vi "Read Network.vi"(8 "error in (no error)":errorcluster, 11 "Sensor Engine Datas in":T1[](array[typedef])) -> (0 "error out":errorcluster, 1 "signal data":dbl[](array[numeric]), 3 "Sensor Engine Datas out":T1[](array[typedef]))   [LabVIEW 2023, in "MM.lvlib"]
uses:
  MM.lvlib
  Sensor Engine Data.ctl
  DataContainer/DataContainer.lvclass
  Shared/Protocol.ctl
  <vilib>/xnet/xnet.llb/XNET Convert (Frame FlexRay to Signal).vi
  Shared/Vires VTD Shared.lvlib
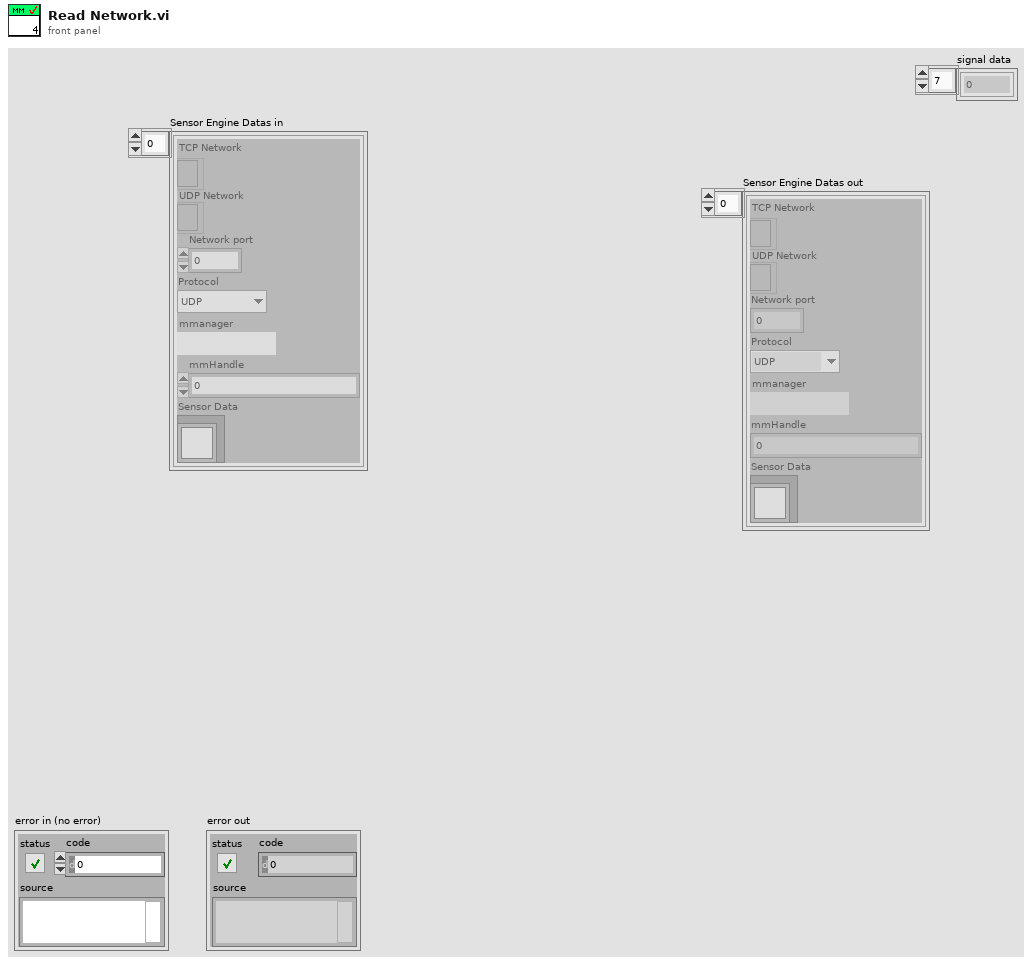
[diagram p1: front panel]
types:
  T1 = typedef "MM.lvlib/Sensor Engine Data.ctl" = cluster{"TCP Network":refnum<k5>, "UDP Network":refnum<k16>, "Network port":i32, "Protocol":T2, "mmanager":path, "mmHandle":u64, "Sensor Data":refnum<class "DataContainer.lvclass">}
  T2 = typedef "Vires VTD Shared.lvlib/Protocol.ctl" = enum16{"UDP", "TCP"}
  T3 = enum16{"Standard", "Buffered", "CRLF", "Immediate"}
  T4 = typedef "XNET Frame FlexRay.ctl" = cluster{"timestamp":timestamp, "payload":u8[], "slot":u16, "type":T5, "cycle count":u8, "startup?":bool, "sync?":bool, "preamble?":bool, "ch A":bool, "ch B":bool, "echo?":bool}
  T5 = typedef "XNET Frame Type FlexRay.ctl" = u8
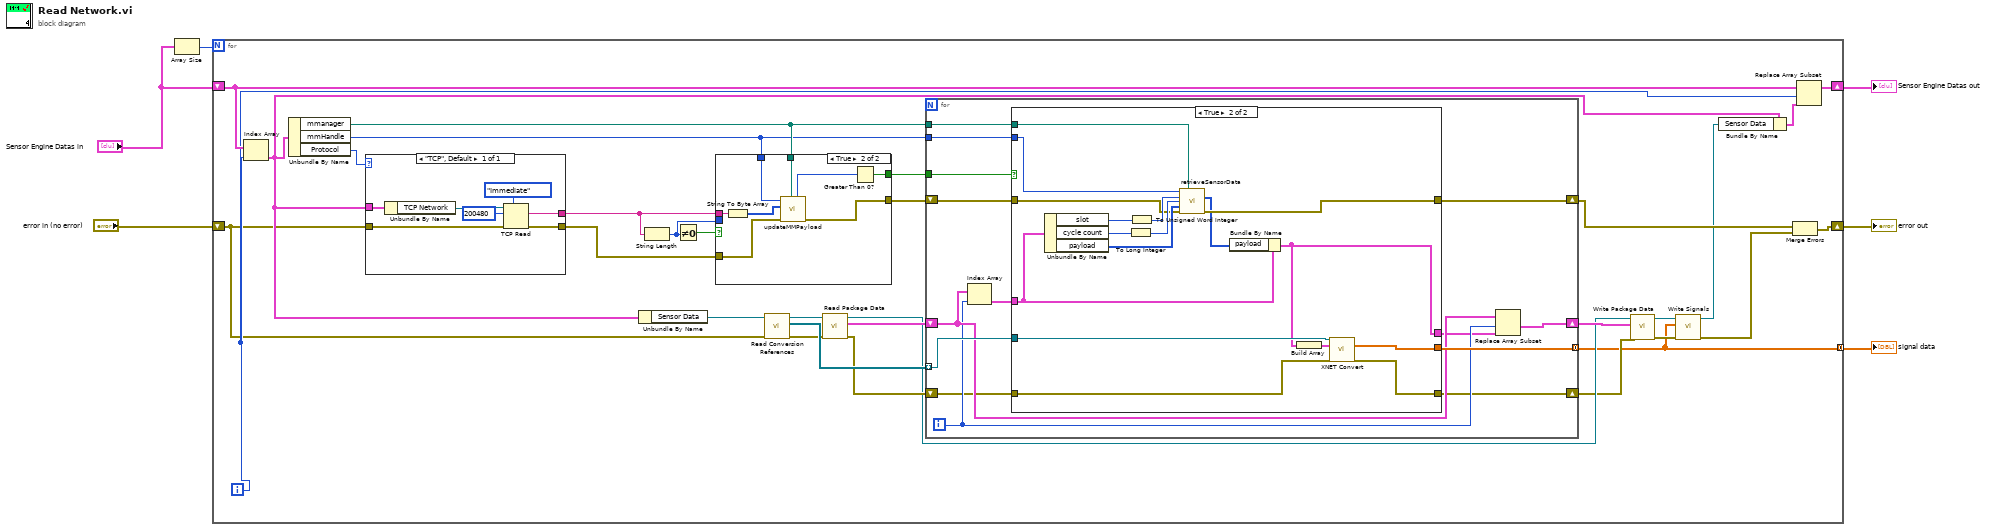
[diagram p0: block diagram]
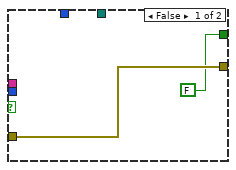
[diagram p3: hidden frame]
diagram:
  n1 = Array Size(array="Sensor Engine Datas in") -> (size(s)=w2:i32)
  n2 = for {
    N: w2 -> [_]
    shift-right: [w15] -> w5
    shift-left: "error in (no error)" -> [w18]
    tunnel: [w7] -> w4 mode=concatenating
    shift-right: [w31] -> w3
    shift-left: "Sensor Engine Datas in" -> [w30]
    i -> [w29]
    n3 = Index Array(array=w30, index=w29) -> (element=w24:T1)
    n4 = Unbundle By Name(w24) -> ("mmanager"=w26:path, "mmHandle"=w25:u64, "Protocol"=w37:T2)
    n5 = case shown="\"TCP\", Default" w37 {
      tunnel: w18 -> [w88]
      tunnel: [w86] -> w34
      tunnel: [w85] -> w27
      tunnel: w24 -> [w83]
      frame "TCP", Default {
        n6 = Unbundle By Name(w83) -> ("TCP Network"=w82:refnum<k5>)
        n7 = TCP Read(connection ID=w82, bytes to read=200480, error in (no error)=w88, 7:T3."Immediate" ("mode (standard)")) -> (data out=w85:string, error out=w86:errorcluster)  [unwired: 1 in, 1 out]
      }
    }
    n8 = Unbundle By Name(w24) -> ("Sensor Data"=w23:refnum<class "DataContainer.lvclass">)
    n9 = String Length(string=w27) -> (length=w36:i32)
    n10 = Not Equal To 0?(x=w36) -> (x != 0?=w35:bool)
    n11 = case shown="True" w35 {
      tunnel: w34 -> [w73 w76]
      tunnel: [w73 w75] -> w33
      tunnel: w27 -> [_ w79]
      tunnel: [FALSE w81] -> w32
      tunnel: w36 -> [_ _]
      tunnel: w26 -> [_ w80]
      tunnel: w25 -> [_ w77]
      frame False {
      }
      frame True {
        n12 = String To Byte Array(string=w79) -> (unsigned byte array=w78:u8[])
        n13 = call "updateMMPayload.vi"("path in"=w80, "error in (no error)"=w76, "payload"=w78, "mmHandle in"=w77) -> ("error out"=w75:errorcluster, "isComplete"=w74:u8)  [unwired: 2 in, 4 out]
        n14 = Greater Than 0?(x=w74) -> (x > 0?=w81:bool)
      }
    }
    n15 = call-dynamic "Read Conversion References.vi"("error in (no error)"=w18, "DataContainer in"=w23) -> ("error out"=w19:errorcluster, "Conversion References"=w20:refnum<k21>[], "DataContainer out"=w22:refnum<class "DataContainer.lvclass">)  [unwired: 7 in]
    n16 = call-dynamic "Read Package Data.vi"("error in (no error)"=w19, "DataContainer in"=w22) -> ("error out"=w17:errorcluster, "Package Data"=w21:T4[], "DataContainer out"=w13:refnum<class "DataContainer.lvclass">)  [unwired: 7 in]
    n17 = for {
      tunnel: w32 -> [w50]
      tunnel: [w48] -> w7 mode=concatenating
      shift-right: [w49] -> w16
      shift-left: w33 -> [w51]
      tunnel: w20 -> [w47] mode=indexing
      shift-right: [w45] -> w14
      shift-left: w21 -> [w44]
      tunnel: w26 -> [w41]
      tunnel: w25 -> [w40]
      shift-right: [w38] -> w12
      shift-left: w17 -> [w39]
      i -> [w43]
      n18 = Index Array(array=w44, index=w43) -> (element=w46:T4)
      n19 = case shown="True" w50 {
        tunnel: w51 -> [w54 w59]
        tunnel: [w54 w58] -> w49
        tunnel: [_ w71] -> w48
        tunnel: w47 -> [_ w69]
        tunnel: w46 -> [w53 w68]
        tunnel: [w53 w65] -> w42
        tunnel: w41 -> [_ w64]
        tunnel: w40 -> [_ w63]
        tunnel: w39 -> [w52 w56]
        tunnel: [w52 w55] -> w38
        frame False {
        }
        frame True {
          n20 = Unbundle By Name(w68) -> ("slot"=w67:u16, "cycle count"=w66:u8, "payload"=w60:u8[])
          n21 = To Long Integer(number=w66) -> (32bit integer=w61:i32)
          n22 = To Unsigned Word Integer(number=w67) -> (unsigned 16bit integer=w62:u16)
          n23 = call "retrieveSensorData.vi"("mmHandle in"=w63, "path in"=w64, "packageID"=w62, "objIndex"=w61, "dataOut"=w60, "error in (no error)"=w59) -> ("dataOut"=w57:u8[], "error out"=w58:errorcluster)  [unwired: 7 in, 1 out]
          n24 = Bundle By Name(cluster=w68, "payload"=w57) -> (w65:T4)
          n25 = Build Array(w65) -> (w70:T4[])
          n26 = call-poly <vilib>:"XNET Convert.vi"("session in"=w69, "frame data"=w70, "error in (no error)"=w56) -> ("signal data"=w71:dbl[], "error out"=w55:errorcluster)  [unwired: 10 in, 1 out]
        }
      }
      n27 = Replace Array Subset(array=w44, new element=w42, index=w43) -> (w45:T4[])
    }
    n28 = call-dynamic "Write Package Data.vi"("error in (no error)"=w12, "Package Data"=w14, "DataContainer in"=w13) -> ("error out"=w10:errorcluster, "DataContainer out"=w11:refnum<class "DataContainer.lvclass">)  [unwired: 7 in]
    n29 = call-dynamic "Write Signals.vi"("error in (no error)"=w10, "Signals"=w7, "DataContainer in"=w11) -> ("error out"=w9:errorcluster, "DataContainer out"=w8:refnum<class "DataContainer.lvclass">)  [unwired: 7 in]
    n30 = Bundle By Name(cluster=w24, "Sensor Data"=w8) -> (w28:T1)
    n31 = Merge Errors(w16, w9) -> (w15:errorcluster)
    n32 = Replace Array Subset(array=w30, new element=w28, index=w29) -> (w31:T1[])
  }
  "error out" <- w5
  "signal data" <- w4
  "Sensor Engine Datas out" <- w3
